vi "levels_to_coupling.vi"(9 "Sensor card":i32=1, 10 "Carrier amplitudes":T1 format="%#_3p", 11 "High carrier amplitudes":T2 format="%#_3p") -> (1 "High at low coupling":cdb[][](array[numeric]), 2 "Low rate coupling":cdb[][](array[numeric]), 3 "High rate couplings":cdb[][][](array[numeric]))   [LabVIEW 2024]
uses:
  main/ilemt_globals.vi
  high_carrier_amplitudes.ctl
  carrier_amplitudes.ctl
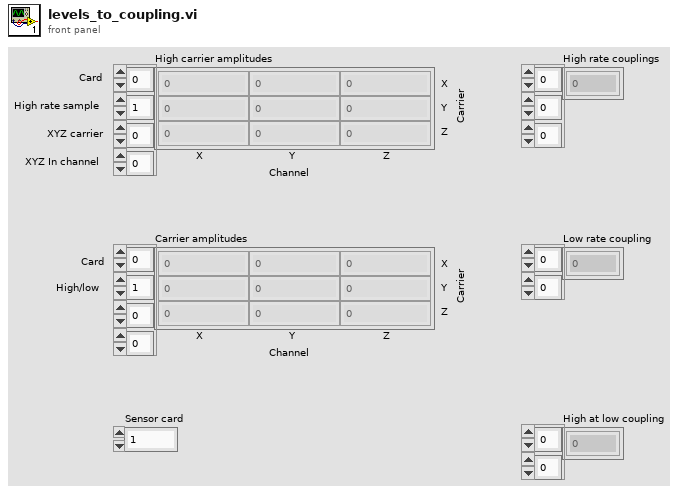
[diagram p1: front panel]
types:
  T1 = typedef "carrier_amplitudes.ctl" = cdb[][][][]
  T2 = typedef "high_carrier_amplitudes.ctl" = cdb[][][][]
  T3 = typedef "coupling_matrix.ctl" = cdb[][]
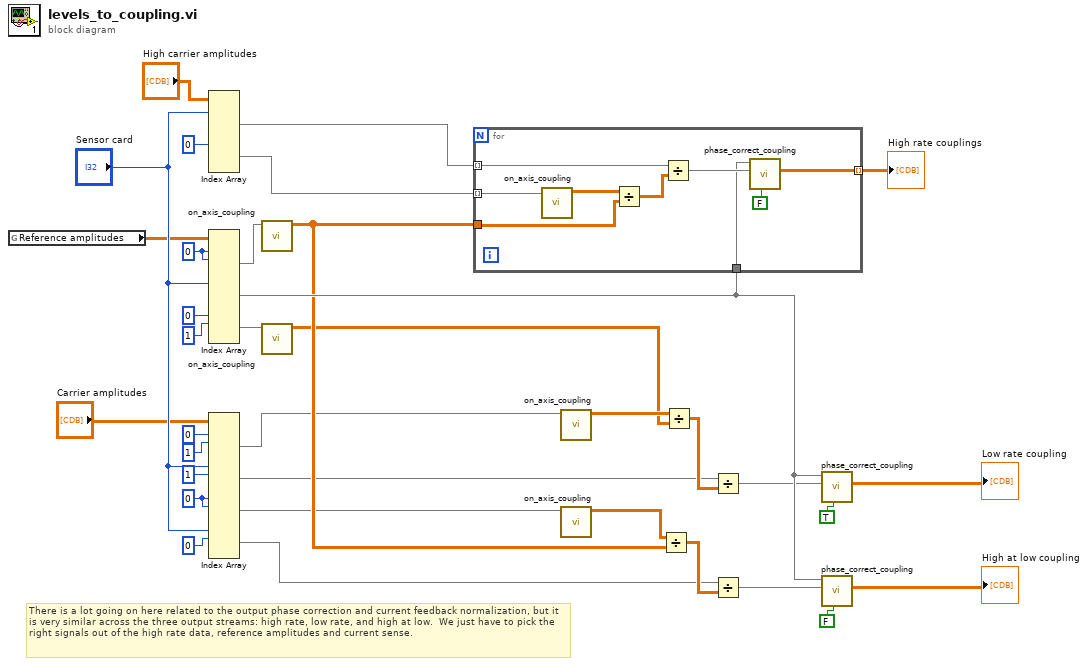
[diagram p0: block diagram]
diagram:
  w22 = 0 ("index (vol)")
  w24 = 0 ("index (vol)")
  # "There is a lot going on here related to the output phase correction and current feedback normalization, but it is very similar across the three output streams: high rate, low rate, and high at low.  We just have to pick the right signals out of the high rate data, reference amplitudes and current sense."
  n1 = global read "ilemt_globals.vi" "Reference amplitudes"() -> (w7:T1)
  n2 = Index Array(array="High carrier amplitudes", index (dim 0) #1="Sensor card", index (dim 0) #2=0 ("index (vol)")) -> (element #1=w32:cdb[][][], element #2=w33:cdb[][][])  [unwired: 6 in]
  n3 = Index Array(array=w7, index (dim 0) #1=w24, index (dim 1) #1=w24, index (dim 0) #2="Sensor card", index (dim 0) #3=0 ("index (vol)"), index (dim 1) #3=1 ("index (page)")) -> (element #1=w6:cdb[][], element #2=w34:cdb[][][], element #3=w11:cdb[][])  [unwired: 7 in]
  n4 = Index Array(array="Carrier amplitudes", index (dim 0) #1=0 ("index (vol)"), index (dim 1) #1=1 ("index (page)"), index (dim 0) #2="Sensor card", index (dim 1) #2=1 ("disabled index (page)"), index (dim 0) #3=w22, index (dim 1) #3=w22, index (dim 0) #4="Sensor card", index (dim 1) #4=0 ("disabled index (page)")) -> (element #1=w16:cdb[][], element #2=w18:cdb[][], element #3=w23:cdb[][], element #4=w21:cdb[][])  [unwired: 8 in]
  n5 = call "on_axis_coupling.vi"("Sense coupling"=w6) -> ("Sense amplitudes"=w31:T3)  [unwired: 10 in]
  n6 = call "on_axis_coupling.vi"("Sense coupling"=w11) -> ("Sense amplitudes"=w17:T3)  [unwired: 10 in]
  n7 = for {
    tunnel: w31 -> [w38]
    tunnel: w32 -> [w40] mode=indexing
    tunnel: w33 -> [w39] mode=indexing
    tunnel: w34 -> [w37]
    tunnel: [w36] -> w35 mode=indexing
    n8 = call "on_axis_coupling.vi"("Sense coupling"=w39) -> ("Sense amplitudes"=w43:T3)  [unwired: 10 in]
    n9 = Divide(x=w43, y=w38) -> (x/y=w44:T3)
    n10 = Divide(x=w40, y=w44) -> (x/y=w42:cdb[][])
    n11 = call "phase_correct_coupling.vi"("Is low?"=FALSE, "Complex coupling"=w42, "Ref carrier ampl"=w37) -> ("Phase corrected coupling"=w36:cdb[][])  [unwired: 7 in, 1 out]
  }
  "High rate couplings" <- w35
  n12 = call "on_axis_coupling.vi"("Sense coupling"=w16) -> ("Sense amplitudes"=w28:T3)  [unwired: 10 in]
  n13 = call "on_axis_coupling.vi"("Sense coupling"=w23) -> ("Sense amplitudes"=w30:T3)  [unwired: 10 in]
  n14 = Divide(x=w30, y=w31) -> (x/y=w29:T3)
  n15 = Divide(x=w28, y=w17) -> (x/y=w27:T3)
  n16 = Divide(x=w18, y=w27) -> (x/y=w19:cdb[][])
  n17 = Divide(x=w21, y=w29) -> (x/y=w20:cdb[][])
  n18 = call "phase_correct_coupling.vi"("Is low?"=TRUE, "Complex coupling"=w19, "Ref carrier ampl"=w34) -> ("Phase corrected coupling"=→"Low rate coupling":cdb[][])  [unwired: 7 in, 1 out]
  n19 = call "phase_correct_coupling.vi"("Is low?"=FALSE, "Complex coupling"=w20, "Ref carrier ampl"=w34) -> ("Phase corrected coupling"=→"High at low coupling":cdb[][])  [unwired: 7 in, 1 out]
